vi "Graphics-HSV to RGB.vi"(0 "Hue":dbl, 7 "Saturation":dbl=1.0, 11 "Value":dbl) -> (4 "Color":u32(colorbox), 6 "Red":u8, 8 "Green":u8, 10 "Blue":u8)   [LabVIEW 2020]
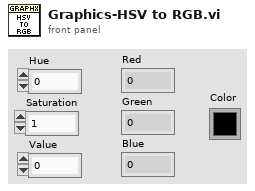
[diagram p1: front panel]
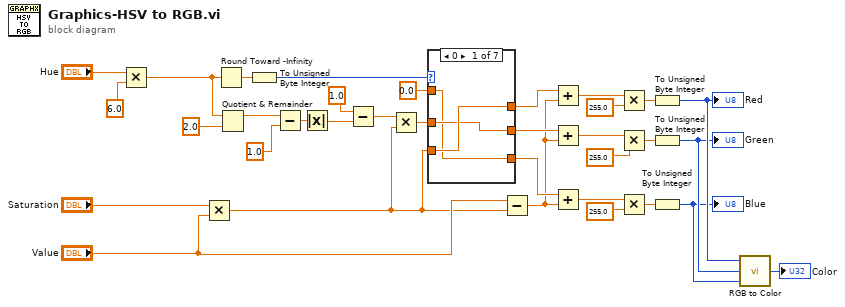
[diagram p0: block diagram]
diagram:
  n1 = Multiply(x="Hue", y=6.0) -> (x*y=w12:dbl)
  n2 = Multiply(x="Saturation", y="Value") -> (x*y=w27:dbl)
  n3 = Round Toward -Infinity(1:w12) -> (0:w30:dbl)
  n4 = Quotient & Remainder(x=w12, y=2.0) -> (x-y*floor(x/y)=w10:dbl)  [unwired: 1 out]
  n5 = To Unsigned Byte Integer(number=w30) -> (unsigned 8bit integer=w13:u8)
  n6 = Subtract(x=w10, y=1.0) -> (x-y=w8:dbl)
  n7 = Absolute Value(x=w8) -> (abs(x)=w7:dbl)
  n8 = Subtract(x=1.0, y=w7) -> (x-y=w5:dbl)
  n9 = Multiply(x=w5, y=w27) -> (x*y=w29:dbl)
  n10 = case shown="0" w13 {
    tunnel: w27 -> [w37 w39 w42 w44 w47 w52 _]
    tunnel: w29 -> [w36 w40 w41 w45 w49 w50 _]
    tunnel: 0.0 -> [w35 w38 w43 w46 w48 w51 w53]
    tunnel: [w37 w40 w43 w46 w49 w52 w53] -> w24
    tunnel: [w36 w39 w42 w45 w48 w51 w53] -> w25
    tunnel: [w35 w38 w41 w44 w47 w50 w53] -> w26
    frame 0 {
    }
    frame 1 {
    }
    frame 2 {
    }
    frame 3 {
    }
    frame 4 {
    }
    frame 5 {
    }
    frame Default {
    }
  }
  n11 = Subtract(x="Value", y=w27) -> (x-y=w23:dbl)
  n12 = Add(x=w24, y=w23) -> (x+y=w14:dbl)
  n13 = Add(x=w25, y=w23) -> (x+y=w15:dbl)
  n14 = Add(x=w26, y=w23) -> (x+y=w16:dbl)
  n15 = Multiply(x=w14, y=255.0) -> (x*y=w21:dbl)
  n16 = Multiply(x=w15, y=255.0) -> (x*y=w20:dbl)
  n17 = Multiply(x=w16, y=255.0) -> (x*y=w18:dbl)
  n18 = To Unsigned Byte Integer(number=w21) -> (unsigned 8bit integer=w4:u8)
  "Red" <- w4
  n19 = To Unsigned Byte Integer(number=w20) -> (unsigned 8bit integer=w3:u8)
  "Green" <- w3
  n20 = To Unsigned Byte Integer(number=w18) -> (unsigned 8bit integer=w2:u8)
  "Blue" <- w2
  n21 = call <vilib>:"RGB to Color.vi"("B"=w2, "G"=w3, "R"=w4) -> ("Color"=→"Color":u32)
